vi "TharConfig.vi"(8 "Error In":errorcluster, 11 "configuration file path":path) -> (0 "Error Out":errorcluster, 1 "serial":string, 2 "current [mA]":u32, 3 "timeout [ms]":u32)   [LabVIEW 2016]
uses:
  <vilib>/Utility/config.llb/Read Key (U32).vi
  <vilib>/Utility/config.llb/Read Key (String).vi
  <vilib>/Utility/config.llb/NI_LVConfig.lvlib
panel:
  out "configuration file path 2":path
  out "appended path":path
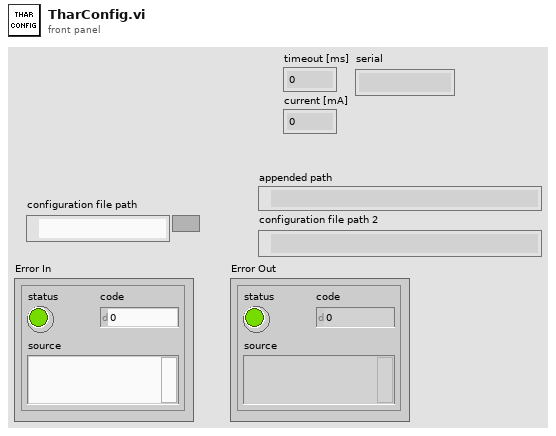
[diagram p1: front panel]
types:
  T1 = typedef "NI_LVConfig.lvlib/Config Data RefNum.ctl" = refnum<k1>
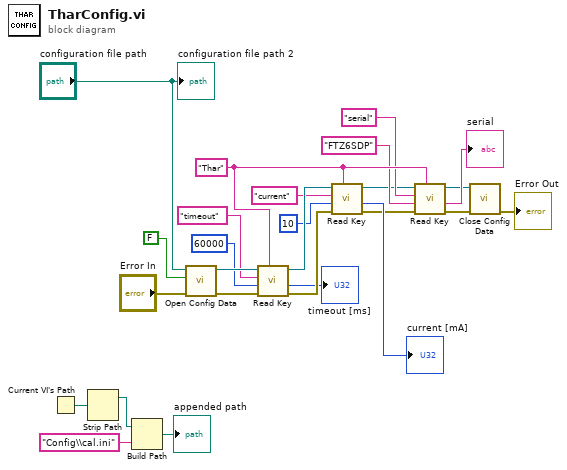
[diagram p0: block diagram]
diagram:
  w14 = "Thar" ("section")
  n1 = Current VI's Path() -> (path=w5:path)
  n2 = Strip Path(path=w5) -> (stripped path=w4:path)  [unwired: 1 out]
  n3 = Build Path(base path=w4, name or relative path="Config\\cal.ini") -> (appended path=→"appended path":path)
  n4 = call <vilib>:"Open Config Data.vi"("error in (no error)"="Error In", "create file if necessary (T)"=FALSE, "configuration file path"="configuration file path") -> ("error out"=w18:errorcluster, "refnum"=w24:T1)  [unwired: 6 in, 1 out]
  n5 = call-poly <vilib>:"Read Key.vi"("section"=w14, "error in (no error)"=w18, "default value"=u32 60000, "key"="timeout" ("element"), "refnum"=w24) -> ("error out"=w19:errorcluster, "value"=→"timeout [ms]":u32, "refnum out"=w23:T1)  [unwired: 3 in, 1 out]
  n6 = call-poly <vilib>:"Read Key.vi"("section"=w14, "error in (no error)"=w19, "default value"=u32 10, "key"="current", "refnum"=w23) -> ("error out"=w13:errorcluster, "value"=→"current [mA]":u32, "refnum out"=w10:T1)  [unwired: 3 in, 1 out]
  n7 = call-poly <vilib>:"Read Key.vi"("section"=w14, "error in (no error)"=w13, "default value"="FTZ6SDP", "key"="serial", "refnum"=w10) -> ("error out"=w8:errorcluster, "value"=→"serial":string, "refnum out"=w6:T1)  [unwired: 3 in, 1 out]
  n8 = call <vilib>:"Close Config Data.vi"("error in (no error)"=w8, "refnum"=w6) -> ("error out"=→"Error Out":errorcluster)  [unwired: 8 in, 1 out]
  "configuration file path 2" <- "configuration file path"
